vi "Find Window.vi"(8 "error in (no error)":errorcluster, 11 "Window Name":string) -> (0 "error out":errorcluster, 3 "Win32 Window Handle":i32)   [LabVIEW 2013, in "Win32 Util.lvlib"]
doc: "This VI calls the FindWindows Function in the User32.dll to obtain the Win32 Window handle for the Window specified by Window Name."
uses:
  Win32 Util.lvlib
  kernel32.dll
  user32.dll
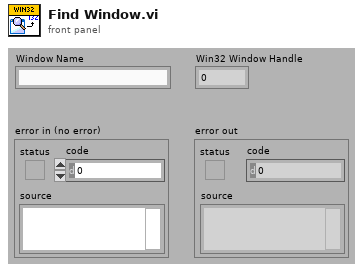
[diagram p1: front panel]
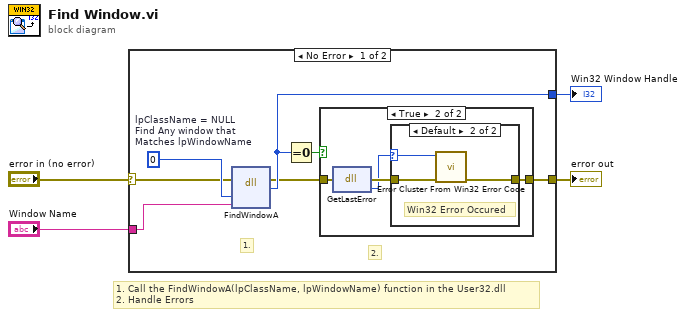
[diagram p0: block diagram]
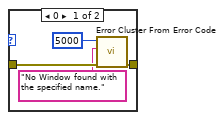
[diagram p3: hidden frame]
diagram:
  # "1. Call the FindWindowA(lpClassName, lpWindowName) function in the User32.dll\n2. Handle Errors"
  n1 = case shown="No Error" "error in (no error)" {
    selector: "error in (no error)" -> [w7 w24]
    tunnel: "Window Name" -> [w10 _]
    tunnel: [w9 _] -> w3
    tunnel: [w8 w24] -> w2
    frame No Error {
      w11 = u32 0  # lpClassName = NULL Find Any window that Matches lpWindowName
      # "2."
      # "1."
      n2 = dll-call lib="user32.dll" fn="FindWindowA"(error in=w7, "lpClassName"=w11, "lpWindowName"=w10) -> (error out=w5:errorcluster, "return type"=w9:i32)  [unwired: 4 in, 1 out]
      n3 = Equal To 0?(x=w9) -> (x = 0?=w6:bool)
      n4 = case shown="True" w6 {
        tunnel: [w12 w16] -> w8
        tunnel: w5 -> [w12 w15]
        frame False {
        }
        frame True {
          n5 = dll-call lib="kernel32.dll" fn="GetLastError" ("user32.dll:FindWindowA")(error in=w15) -> (error out=w14:errorcluster, "return type"=w13:i32)  [unwired: 2 in, 1 out]
          n6 = case shown="Default" w13 {
            selector: w13 -> [_ w21]
            tunnel: [w20 w23] -> w16
            tunnel: w14 -> [w19 w22]
            frame 0 {
              n7 = call <vilib>:"Error Cluster From Error Code.vi"("error in (no error)"=w19, "error message (\"\")"="No Window found with the specified name." ("error message (\"\")"), "error code (0)"=5000) -> ("error out"=w20:errorcluster)  [unwired: 6 in]
            }
            frame Default {
              # "Win32 Error Occured"
              n8 = call "Error Cluster From Win32 Error Code.vi"("error in (no error)"=w22, "error code (0)"=w21) -> ("error out"=w23:errorcluster)  [unwired: 9 in]
            }
          }
        }
      }
    }
    frame Error {
    }
  }
  "error out" <- w2
  "Win32 Window Handle" <- w3
